vi "MALT132 Get One.vi"(8 "error in":errorcluster, 9 "port":i32, 10 "address":i32) -> (0 "error out":errorcluster, 3 "status":bool)   [LabVIEW 2018]
uses:
  Types/MALT CardTypes.ctl
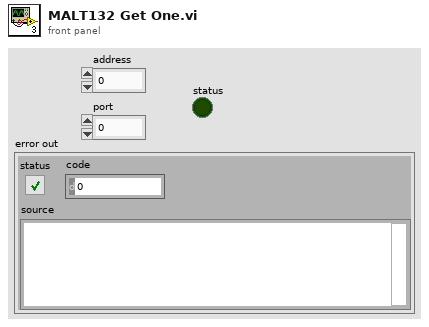
[diagram p1: front panel]
types:
  T1 = typedef "MALT CardTypes.ctl" = enum32{"-", "YAV90832", "YAV904X8", "MALT132", "YAV91616", "YAV90PIN", "YAV90096", "YAV90HVT", "YAV90CLR", "YAV90128", "YAV90PNE", "YAVCANCON", "YAV91775", "YAV90XXX", "YAV90MMU", "H730050", "H710060", "H710061", "YAV90304", "MMI", "YAV90060", "YAV90MUX", "YAV90059", "Not Defined"}
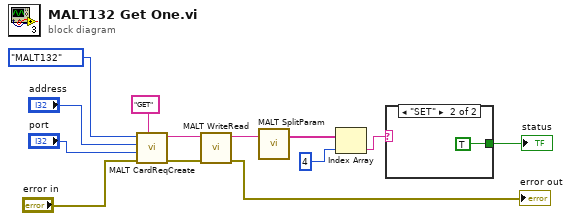
[diagram p0: block diagram]
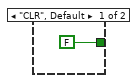
[diagram p2: hidden frame]
diagram:
  n1 = call "MALT CardReqCreate.vi"("Cmd"="GET" ("cmd"), "error in"="error in", "Port"="port", "Address"="address", "CardType"=MALT_CardTypes."MALT132" ("MALT CardType")) -> ("error out"=w3:errorcluster, "request"=w7:string)  [unwired: 5 in]
  n2 = call "MALT WriteRead.vi"("error in"=w3, "Request"=w7) -> ("error out"=→"error out":errorcluster, "Response"=w13:string)  [unwired: 8 in]
  n3 = call "MALT SplitParam.vi"("Line"=w13) -> ("Items"=w11:string[])  [unwired: 2 in]
  n4 = Index Array(array=w11, index=4) -> (element=w9:string)
  n5 = case shown="\"SET\"" w9 {
    tunnel: [FALSE TRUE] -> w8
    frame "CLR", Default {
    }
    frame "SET" {
    }
  }
  "status" <- w8
